vi "UDP Query.vi"(7 "timeout, ms (5000)":i32=5000, 8 "error in (no error)":errorcluster, 9 "port (53)":u16=53, 10 "address":string="8.8.8.8", 11 "request":T2 {"header"."opcode" items=["Query"=0, "IQuery"=1, "Status"=2, "Notify"=4, "Update"=5, "DSO"=6]; "questions"."class" items=["IN"=1, "CH"=3, "HS"=4, "NONE"=254, "*"=255]; "questions"."type" items=["A"=1, "NS"=2, "MD"=3, "MF"=4, "CNAME"=5, "SOA"=6, "MB"=7, "MG"=8, "MR"=9, "NULL"=10, "WKS"=11, "PTR"=12, "HINFO"=13, "MINFO"=14, "MX"=15, "TXT"=16, "RP"=17, "AFSDB"=18, "X25"=19, "ISDN"=20, "RT"=21, "NSAP"=22, "NSAP-PTR"=23, "SIG"=24, "KEY"=25, "PX"=26, "GPOS"=27, "AAAA"=28, "LOC"=29, "NXT"=30, "EID"=31, "NIMLOC"=32, "SRV"=33, "ATMA"=34, "NAPTR"=35, "KX"=36, "CERT"=37, "A6"=38, "DNAME"=39, "SINK"=40, "OPT"=41, "APL"=42, "DS"=43, "SSHFP"=44, "IPSECKEY"=45, "RRSIG"=46, "NSEC"=47, "DNSKEY"=48, "DHCID"=49, "NSEC3"=50, "NSEC3PARAM"=51, "TLSA"=52, "SMIMEA"=53, "HIP"=55, "NINFO"=56, "RKEY"=57, "TALINK"=58, "CDS"=59, "CDNSKEY"=60, "OPENPGPKEY"=61, "CSYNC"=62, "ZONEMD"=63, "SVCB"=64, "HTTPS"=65, "SPF"=99, "UINFO"=100, "UID"=101, "GID"=102, "UNSPEC"=103, "NID"=104, "L32"=105, "L64"=106, "LP"=107, "EUI48"=108, "EUI64"=109, "TKEY"=249, "TSIG"=250, "IXFR"=251, "AXFR"=252, "MAILB"=253, "MAILA"=254, "*"=255, "URI"=256, "CAA"=257, "AVC"=258, "DOA"=259, "AMTRELAY"=260, "TA"=32768, "DLV"=32769]}) -> (0 "error out":errorcluster)   [LabVIEW 2015, in "PL DNS Client.lvlib"]
doc: "Sends DNS query over UDP to specified <b>address</b> and <b>port</b> and parses received response."
uses:
  PL DNS Client.lvlib
panel:
  out "response":T1 {"header"."response code" items=["NoError"=0, "FormErr"=1, "ServFail"=2, "NXDomain"=3, "NotImp"=4, "Refused"=5, "YXDomain"=6, "YXRRSet"=7, "NXRRSet"=8, "NotAuth"=9, "NotZone"=10, "DSOTYPENI"=11, "BADVERS/BADSIG"=16, "BADKEY"=17, "BADTIME"=18, "BADMODE"=19, "BADNAME"=20, "BADALG"=21, "BADTRUNC"=22, "BADCOOKIE"=23]; "header"."opcode" items=["Query"=0, "IQuery"=1, "Status"=2, "Notify"=4, "Update"=5, "DSO"=6]; "additional records"."class" items=["IN"=1, "CH"=3, "HS"=4]; "additional records"."type" items=["A"=1, "NS"=2, "MD"=3, "MF"=4, "CNAME"=5, "SOA"=6, "MB"=7, "MG"=8, "MR"=9, "NULL"=10, "WKS"=11, "PTR"=12, "HINFO"=13, "MINFO"=14, "MX"=15, "TXT"=16, "RP"=17, "AFSDB"=18, "X25"=19, "ISDN"=20, "RT"=21, "NSAP"=22, "NSAP-PTR"=23, "SIG"=24, "KEY"=25, "PX"=26, "GPOS"=27, "AAAA"=28, "LOC"=29, "NXT"=30, "EID"=31, "NIMLOC"=32, "SRV"=33, "ATMA"=34, "NAPTR"=35, "KX"=36, "CERT"=37, "A6"=38, "DNAME"=39, "SINK"=40, "OPT"=41, "APL"=42, "DS"=43, "SSHFP"=44, "IPSECKEY"=45, "RRSIG"=46, "NSEC"=47, "DNSKEY"=48, "DHCID"=49, "NSEC3"=50, "NSEC3PARAM"=51, "TLSA"=52, "SMIMEA"=53, "HIP"=55, "NINFO"=56, "RKEY"=57, "TALINK"=58, "CDS"=59, "CDNSKEY"=60, "OPENPGPKEY"=61, "CSYNC"=62, "ZONEMD"=63, "SVCB"=64, "HTTPS"=65, "SPF"=99, "UINFO"=100, "UID"=101, "GID"=102, "UNSPEC"=103, "NID"=104, "L32"=105, "L64"=106, "LP"=107, "EUI48"=108, "EUI64"=109, "URI"=256, "CAA"=257, "AVC"=258, "DOA"=259, "AMTRELAY"=260, "TA"=32768, "DLV"=32769]; "authority records"."class" items=["IN"=1, "CH"=3, "HS"=4]; "authority records"."type" items=["A"=1, "NS"=2, "MD"=3, "MF"=4, "CNAME"=5, "SOA"=6, "MB"=7, "MG"=8, "MR"=9, "NULL"=10, "WKS"=11, "PTR"=12, "HINFO"=13, "MINFO"=14, "MX"=15, "TXT"=16, "RP"=17, "AFSDB"=18, "X25"=19, "ISDN"=20, "RT"=21, "NSAP"=22, "NSAP-PTR"=23, "SIG"=24, "KEY"=25, "PX"=26, "GPOS"=27, "AAAA"=28, "LOC"=29, "NXT"=30, "EID"=31, "NIMLOC"=32, "SRV"=33, "ATMA"=34, "NAPTR"=35, "KX"=36, "CERT"=37, "A6"=38, "DNAME"=39, "SINK"=40, "OPT"=41, "APL"=42, "DS"=43, "SSHFP"=44, "IPSECKEY"=45, "RRSIG"=46, "NSEC"=47, "DNSKEY"=48, "DHCID"=49, "NSEC3"=50, "NSEC3PARAM"=51, "TLSA"=52, "SMIMEA"=53, "HIP"=55, "NINFO"=56, "RKEY"=57, "TALINK"=58, "CDS"=59, "CDNSKEY"=60, "OPENPGPKEY"=61, "CSYNC"=62, "ZONEMD"=63, "SVCB"=64, "HTTPS"=65, "SPF"=99, "UINFO"=100, "UID"=101, "GID"=102, "UNSPEC"=103, "NID"=104, "L32"=105, "L64"=106, "LP"=107, "EUI48"=108, "EUI64"=109, "URI"=256, "CAA"=257, "AVC"=258, "DOA"=259, "AMTRELAY"=260, "TA"=32768, "DLV"=32769]; "answers"."class" items=["IN"=1, "CH"=3, "HS"=4]; "answers"."type" items=["A"=1, "NS"=2, "MD"=3, "MF"=4, "CNAME"=5, "SOA"=6, "MB"=7, "MG"=8, "MR"=9, "NULL"=10, "WKS"=11, "PTR"=12, "HINFO"=13, "MINFO"=14, "MX"=15, "TXT"=16, "RP"=17, "AFSDB"=18, "X25"=19, "ISDN"=20, "RT"=21, "NSAP"=22, "NSAP-PTR"=23, "SIG"=24, "KEY"=25, "PX"=26, "GPOS"=27, "AAAA"=28, "LOC"=29, "NXT"=30, "EID"=31, "NIMLOC"=32, "SRV"=33, "ATMA"=34, "NAPTR"=35, "KX"=36, "CERT"=37, "A6"=38, "DNAME"=39, "SINK"=40, "OPT"=41, "APL"=42, "DS"=43, "SSHFP"=44, "IPSECKEY"=45, "RRSIG"=46, "NSEC"=47, "DNSKEY"=48, "DHCID"=49, "NSEC3"=50, "NSEC3PARAM"=51, "TLSA"=52, "SMIMEA"=53, "HIP"=55, "NINFO"=56, "RKEY"=57, "TALINK"=58, "CDS"=59, "CDNSKEY"=60, "OPENPGPKEY"=61, "CSYNC"=62, "ZONEMD"=63, "SVCB"=64, "HTTPS"=65, "SPF"=99, "UINFO"=100, "UID"=101, "GID"=102, "UNSPEC"=103, "NID"=104, "L32"=105, "L64"=106, "LP"=107, "EUI48"=108, "EUI64"=109, "URI"=256, "CAA"=257, "AVC"=258, "DOA"=259, "AMTRELAY"=260, "TA"=32768, "DLV"=32769]}
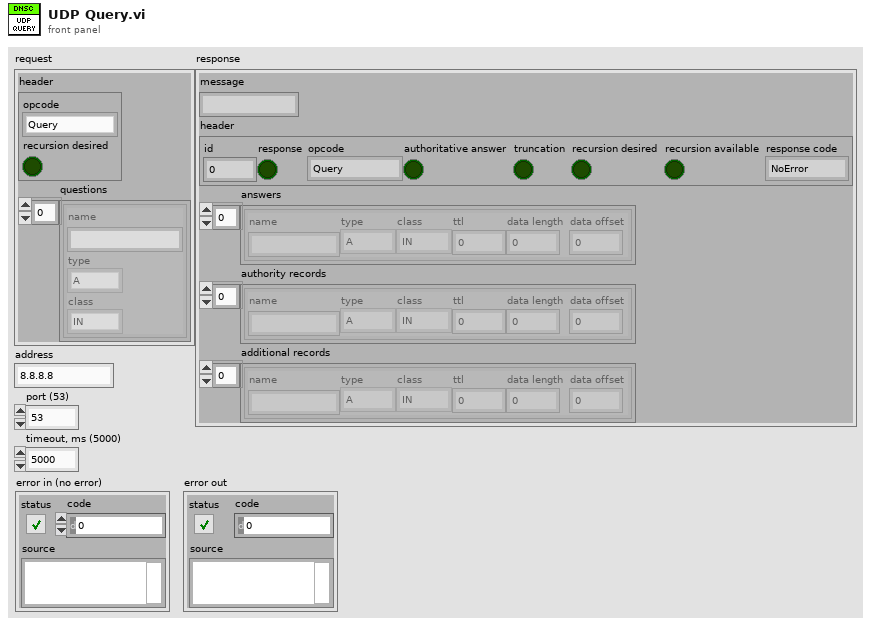
[diagram p1: front panel]
types:
  T1 = cluster{"message":string, "header":cluster{"id":u16, "response":bool, "opcode":u8, "authoritative answer":bool, "truncation":bool, "recursion desired":bool, "recursion available":bool, "response code":u16}, "answers":cluster{"name":string, "type":u16, "class":u16, "ttl":u32, "data length":u16, "data offset":u16}[], "authority records":cluster{"name":string, "type":u16, "class":u16, "ttl":u32, "data length":u16, "data offset":u16}[], "additional records":cluster{"name":string, "type":u16, "class":u16, "ttl":u32, "data length":u16, "data offset":u16}[]}
  T2 = cluster{"header":cluster{"opcode":u8, "recursion desired":bool}, "questions":cluster{"name":string, "type":u16, "class":u16}[]}
  T3 = cluster{"name":string, "type":u16, "class":u16}[]
  T4 = cluster{u16, "opcode":u8, "recursion desired":bool}
  T5 = cluster{cluster{u16, "opcode":u8, "recursion desired":bool}, "questions":cluster{"name":string, "type":u16, "class":u16}[]}
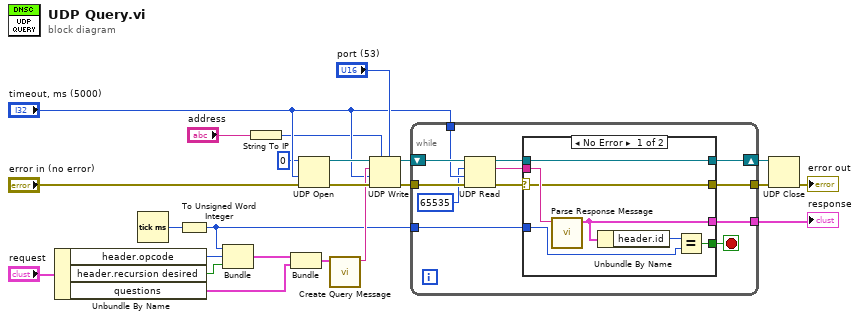
[diagram p0: block diagram]
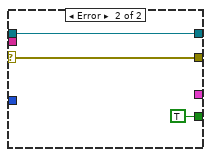
[diagram p2: hidden frame]
diagram:
  n1 = Unbundle By Name("request") -> ("header.opcode"=w12:u8, "header.recursion desired"=w13:bool, "questions"=w8:T3)
  n2 = Tick Count (ms)() -> (millisecond timer value=w6:u32)
  n3 = To Unsigned Word Integer(number=w6) -> (unsigned 16bit integer=w5:u16)
  n4 = Bundle(w5, "opcode"=w12, "recursion desired"=w13) -> (w9:T4)  [unwired: 1 in]
  n5 = String To IP(1:"address") -> (0:w3:u32)
  n6 = Bundle(w9, "questions"=w8) -> (w7:T5)  [unwired: 1 in]
  n7 = UDP Open(8:"error in (no error)", 9:"timeout, ms (5000)", 11:u16 0 ("port")) -> (port=w22:refnum<k16>, 0:w23:errorcluster)  [unwired: 2 in, 1 out]
  n8 = call "Create Query Message.vi"("query"=w7) -> ("message"=w11:string)  [unwired: 10 in]
  n9 = UDP Write(address=w3, port or service name="port (53)", connection ID=w22, data in=w11, 8:w23, 9:"timeout, ms (5000)") -> (error out=w19:errorcluster, 3:w20:refnum<k16>)
  n10 = while {
    tunnel: w19 -> [w29]
    tunnel: "timeout, ms (5000)" -> [w34]
    shift-right: [w30] -> w18
    shift-left: w20 -> [w35]
    tunnel: [w33] -> w2
    tunnel: [w28] -> w15
    tunnel: w5 -> [w27]
    stop <- w25 stop-if-true
    n11 = UDP Read(connection ID=w35, max size (548)=65535, timeout ms (25000)=w34, 8:w29) -> (data out=w32:string, error out=w26:errorcluster, 3:w31:refnum<k16>)  [unwired: 2 out]
    n12 = case shown="No Error" w26 {
      selector: w26 -> [w38 w44]
      tunnel: [w40 _] -> w33
      tunnel: w32 -> [w41 _]
      tunnel: [w39 TRUE] -> w25
      tunnel: w31 -> [w42 w45]
      tunnel: [w42 w45] -> w30
      tunnel: [w38 w44] -> w28
      tunnel: w27 -> [w36 _]
      frame No Error {
        n13 = call "Parse Response Message.vi"("message"=w41) -> ("response"=w40:T1)  [unwired: 10 in]
        n14 = Unbundle By Name(w40) -> ("header.id"=w37:u16)
        n15 = Equal?(x=w37, y=w36) -> (x = y?=w39:bool)
      }
      frame Error {
      }
    }
  }
  "response" <- w2
  n16 = UDP Close(connection ID=w18, 8:w15) -> (error out=→"error out":errorcluster)  [unwired: 1 out]
